vi "Is Error.vi"(11 "Base Event in":refnum<class "Base Event.lvclass">) -> (3 "Base Event out":refnum<class "Base Event.lvclass">)   [LabVIEW 2021, in "jettl.lvlib" / "Base Event.lvlib" / "Base Event.lvclass"]
uses:
  Base Event.lvclass
  State/Error State/Error State.lvclass
  C:/git/jettl/src/jettl/Base Event/State/State/State.lvclass
  Base Event.lvclass/Base Event.ctl
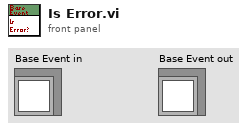
[diagram p1: front panel]
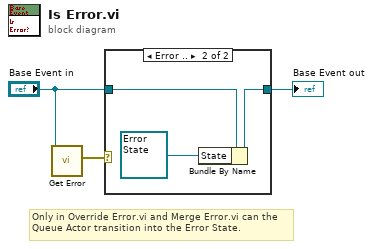
[diagram p0: block diagram]
diagram:
  # "Only in Override Error.vi and Merge Error.vi can the Queue Actor transition into the Error State."
  n1 = call-dynamic "Get Error.vi"("Base Event in"="Base Event in") -> ("Error"=w1:errorcluster)  [unwired: 10 in]
  n2 = case shown="Error .." w1 {
    tunnel: [w4 w6] -> w3
    tunnel: "Base Event in" -> [w4 w7]
    frame No Error {
    }
    frame Error {
      n3 = Bundle By Name(cluster=w7, "State"=refnum<class "Error State.lvclass"> refnum ("jettl.lvlib:Error Event State.lvclass")) -> (w6:refnum<class "Base Event.lvclass">)
    }
  }
  "Base Event out" <- w3
